vi "Create MeasData Q.vi"(8 "error in (no error)":errorcluster, 10 "MeasurementData":T1, 11 "QName":string) -> (0 "error out":errorcluster, 3 "MeasDataQRef":refnum<queue>)   [LabVIEW 2020]
doc: "Developed by Kevin Thompson\nThompson Engineering, LLC\nkevin@thompsonengineering.net"
uses:
  TD MeasData--cluster.ctl
  GBL DataQ Ref.vi
panel:
  out "data reference":u32
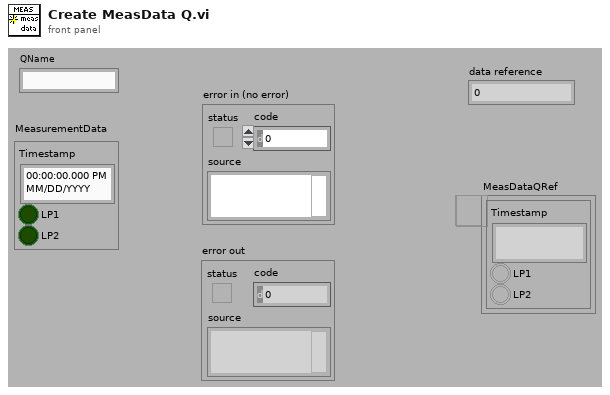
[diagram p1: front panel]
types:
  T1 = typedef "TD MeasData--cluster.ctl" = cluster{"Timestamp":timestamp, "LP1":bool, "LP2":bool}
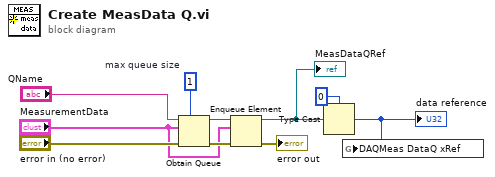
[diagram p0: block diagram]
diagram:
  w9 = 1  # max queue size
  n1 = Obtain Queue(max queue size (-1, unlimited)=w9, name (unnamed)="QName", element data type="MeasurementData", error in (no error)="error in (no error)") -> (queue out=w6:refnum<queue>, error out=w7:errorcluster)  [unwired: 1 in, 1 out]
  n2 = Enqueue Element(queue=w6, element="MeasurementData", error in (no error)=w7) -> (queue out=w3:refnum<queue>, error out=→"error out":errorcluster)  [unwired: 1 in, 1 out]
  "MeasDataQRef" <- w3
  n3 = Type Cast(type=u32 0, x=w3) -> (*(type *) &x=w1:u32)
  "data reference" <- w1
  n4 = global write "GBL DataQ Ref.vi" "DAQMeas DataQ xRef"(w1) -> ()
